vi "vectorAddingSwerve.vi"(8 "LeftX":dbl format="%#_13g", 11 "LeftY":dbl) -> (0 "FinalAngle":dbl, 3 "FinalVelocity":dbl)   [LabVIEW 2020]
panel:
  # "<-- This is Speed Straight"
  # "<-- This is Speed Angled"
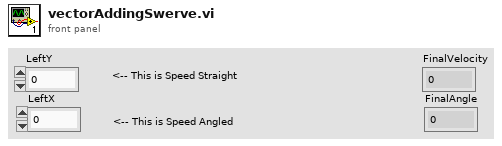
[diagram p1: front panel]
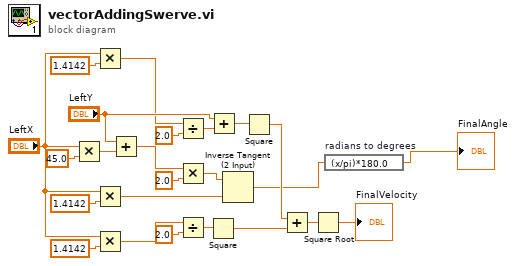
[diagram p0: block diagram]
diagram:
  n1 = Multiply(x="LeftX", y=45.0) -> (x*y=w23:dbl)
  n2 = Multiply(x="LeftX", y=1.4142) -> (x*y=w17:dbl)
  n3 = Multiply(x="LeftX", y=1.4142) -> (x*y=w3:dbl)
  n4 = Multiply(x="LeftX", y=1.4142) -> (x*y=w9:dbl)
  n5 = Add(x="LeftY", y=w23) -> (x+y=w22:dbl)
  n6 = Divide(x=w17, y=2.0) -> (x/y=w15:dbl)
  n7 = Multiply(x=w22, y=2.0) -> (x*y=w4:dbl)
  n8 = Divide(x=w9, y=2.0) -> (x/y=w7:dbl)
  n9 = Square(x=w7) -> (x^2=w12:dbl)
  n10 = Add(x="LeftY", y=w15) -> (x+y=w14:dbl)
  n11 = Inverse Tangent (2 Input)(1:w3, 2:w4) -> (0:w2:dbl)
  n12 = Square(x=w14) -> (x^2=w13:dbl)
  n13 = Add(x=w13, y=w12) -> (x+y=w6:dbl)
  n14 = Square Root(x=w6) -> (sqrt(x)=→"FinalVelocity":dbl)
  n15 = expression code="(x/pi)*180.0" "radians to degrees"(w2) -> (→"FinalAngle":dbl)
